vi "CheckForFileExists.vi"(0 "Path":path, 11 "error in":errorcluster) -> (4 "Dup Path":path, 8 "File Exists?":bool, 15 "error out":errorcluster)   [LabVIEW 2016, in "Drona.lvlib"]
uses:
  Drona.lvlib
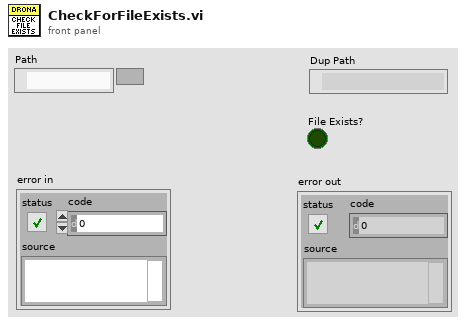
[diagram p1: front panel]
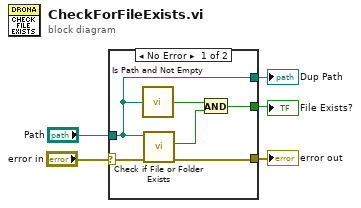
[diagram p0: block diagram]
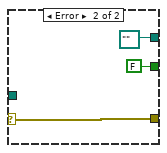
[diagram p2: hidden frame]
diagram:
  n1 = case shown="No Error" "error in" {
    selector: "error in" -> [w11 w14]
    tunnel: "Path" -> [w9 _]
    tunnel: [w9 path "" ("dup path")] -> w2
    tunnel: [w10 w14] -> w3
    tunnel: [w6 FALSE] -> w1
    frame No Error {
      n2 = call <vilib>:"Is Path and Not Empty.vi"("path"=w9) -> ("Is Path and Not Empty?"=w7:bool)  [unwired: 4 in]
      n3 = call <vilib>:"Check if File or Folder Exists.vi"("error in (no error)"=w11, "path"=w9) -> ("error out"=w10:errorcluster, "file or folder exists?"=w8:bool)  [unwired: 7 in, 1 out]
      n4 = And(x=w7, y=w8) -> (x .and. y?=w6:bool)
    }
    frame Error {
    }
  }
  "error out" <- w3
  "Dup Path" <- w2
  "File Exists?" <- w1
